vi "Keyence LJ-V7000 Configure.vi"() -> ()   [LabVIEW 2014]
doc: "This example indicates how to change settings of the controller."
uses:
  Public/constant/Comm Interface.ctl
  Public/Clusters/Ethernet Config.ctl
  Public/constant/Setting Depth.ctl
  Public/Clusters/Target Setting.ctl
  Public/constant/Setting Type.ctl
  State Machine State3.ctl
  Keyence LJ-V7000.lvlib
panel:
  out "Accessing \nthe SAVE area":bool
  out "Accessing the SAVE area":bool
  in  "Depth":T1=1 items=["WRITE AREA", "RUNNING AREA", "SAVE AREA"]
  out "Setting Error":u32
  in  "Depth":T1 items=["WRITE AREA", "RUNNING AREA", "SAVE AREA"]
  out "Setting Data":u8[](array[numeric])
  in  "Data Size":u32
  in  "Target Setting":T2={"Type"=1, "Category"=0, "Item"=0, "Target 1"=0, "Target 2"=0, "Target 3"=0, "Target 4"=0} {"Type" items=["ENVIRONMENT"=1, "COMMON MEASUREMENT"=2, "PROGRAM 0"=16, "PROGRAM 1"=17, "PROGRAM 2"=18, "PROGRAM 3"=19, "PROGRAM 4"=20, "PROGRAM 5"=21, "PROGRAM 6"=22, "PROGRAM 7"=23, "PROGRAM 8"=24, "PROGRAM 9"=25, "PROGRAM 10"=26, "PROGRAM 11"=27, "PROGRAM 12"=28, "PROGRAM 13"=29, "PROGRAM 14"=30, "PROGRAM 15"=31]}
  in  "Depth":T1 items=["WRITE AREA", "RUNNING AREA", "SAVE AREA"]
  out "Setting Error":u32
  in  "Setting Data":u8[](array[numeric])
  in  "Target Setting":T2={"Type"=1, "Category"=0, "Item"=0, "Target 1"=0, "Target 2"=0, "Target 3"=0, "Target 4"=0} {"Type" items=["ENVIRONMENT"=1, "COMMON MEASUREMENT"=2, "PROGRAM 0"=16, "PROGRAM 1"=17, "PROGRAM 2"=18, "PROGRAM 3"=19, "PROGRAM 4"=20, "PROGRAM 5"=21, "PROGRAM 6"=22, "PROGRAM 7"=23, "PROGRAM 8"=24, "PROGRAM 9"=25, "PROGRAM 10"=26, "PROGRAM 11"=27, "PROGRAM 12"=28, "PROGRAM 13"=29, "PROGRAM 14"=30, "PROGRAM 15"=31]}
  in  "Depth":T1 items=["WRITE AREA", "RUNNING AREA", "SAVE AREA"]
  in  "Update Write Settings Area":bool
  in  "Reflect Setting":bool
  in  "Get Setting":bool
  in  "Set Setting":bool
  in  "Stop VI":bool
  in  "Ethernet Config":T4={"IP Address"=[192, 168, 0, 1], "Port No"=24691}
  in  "Comm Interface":T5
  # "Reflect Settings in the\nWRITE Settings Area"
  # "Communication Configuration"
  # "Set Setting"
  # "Get Setting"
  # "Update WRITE Settings Area"
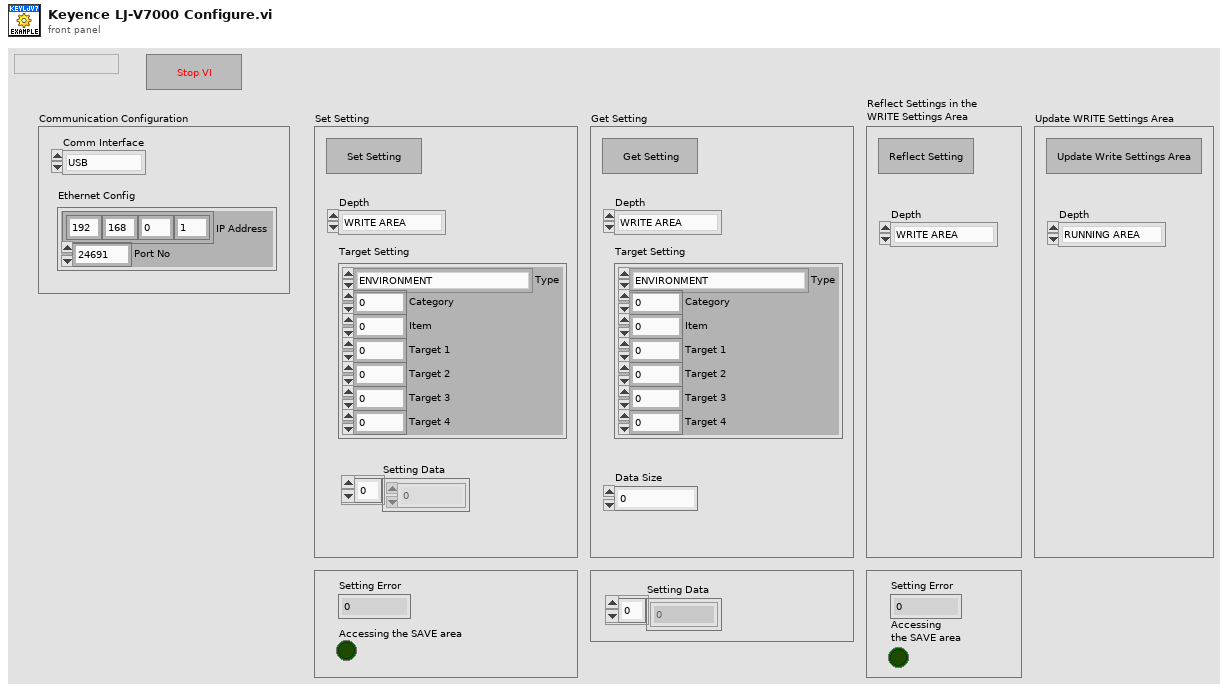
[diagram p1: front panel]
types:
  T1 = typedef "Keyence LJ-V7000.lvlib/Setting Depth.ctl" = u8
  T2 = typedef "Keyence LJ-V7000.lvlib/Target Setting.ctl" = cluster{"Type":T3, "Category":u8, "Item":u8, "Target 1":u8, "Target 2":u8, "Target 3":u8, "Target 4":u8}
  T3 = typedef "Keyence LJ-V7000.lvlib/Setting Type.ctl" = u8
  T4 = typedef "Keyence LJ-V7000.lvlib/Ethernet Config.ctl" = cluster{"IP Address":u8[], "Port No":u16}
  T5 = typedef "Keyence LJ-V7000.lvlib/Comm Interface.ctl" = enum8{"USB", "ETHERNET"}
  T6 = typedef "State Machine State3.ctl" = enum16{"Idle", "Set Setting", "Get Setting", "Reflect Setting", "Update Write Settings Area"}
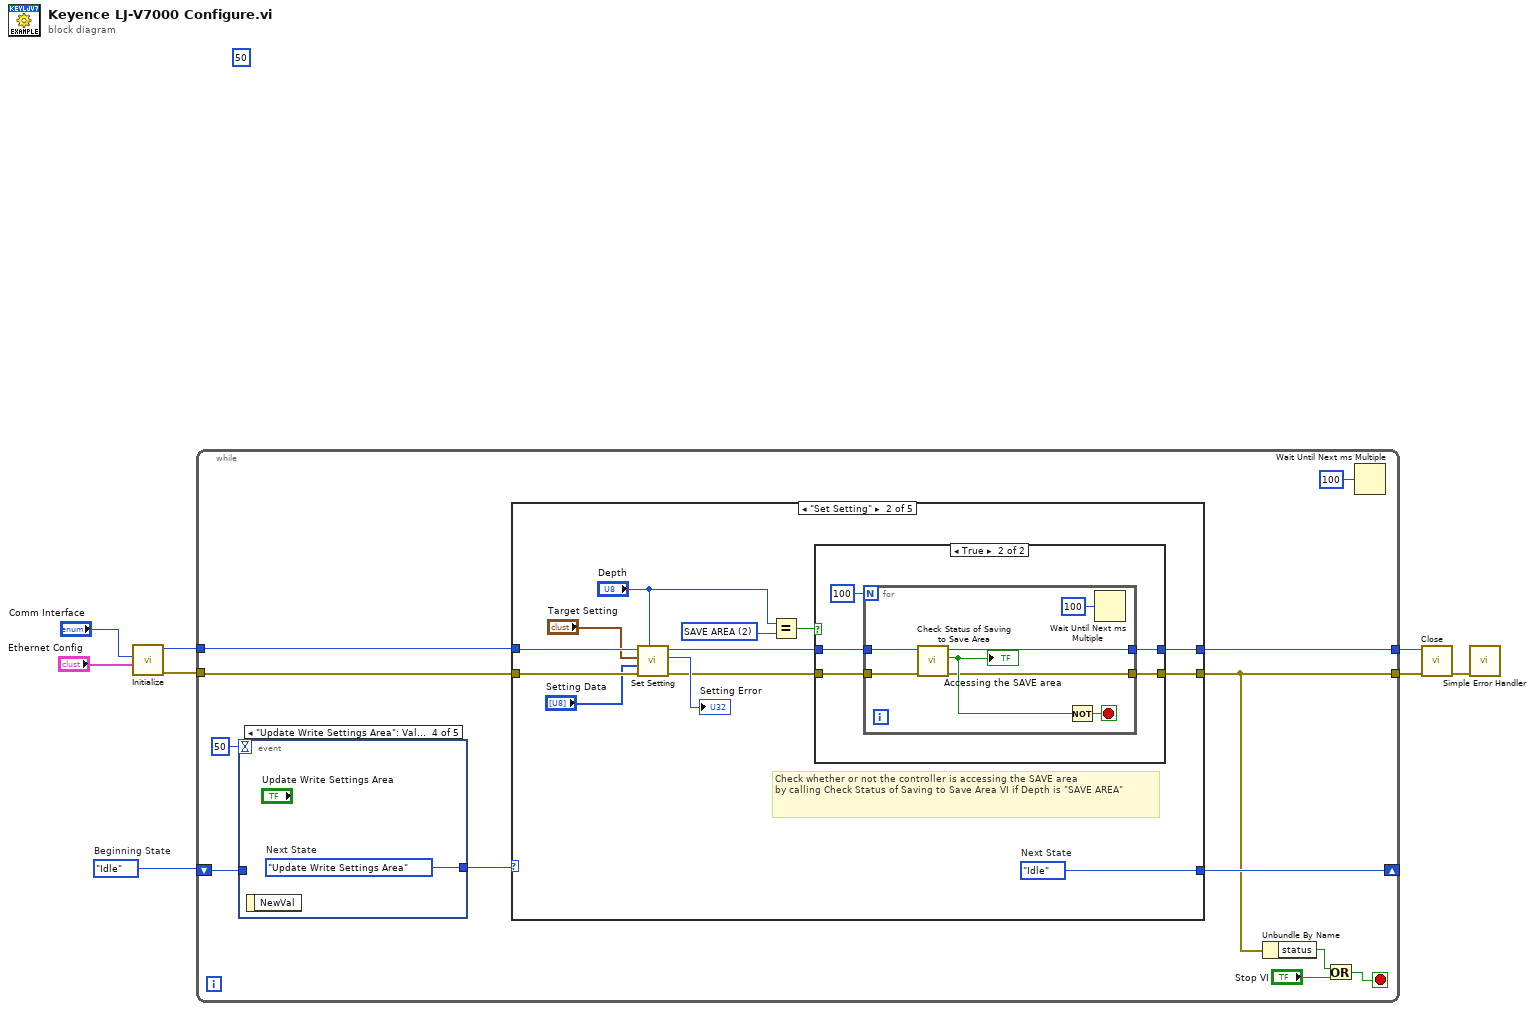
[diagram p0: block diagram]
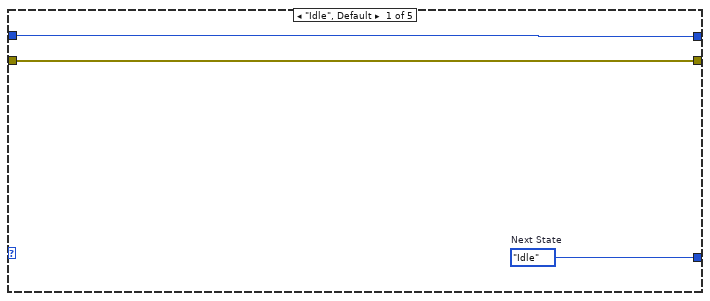
[diagram p2: hidden frame]
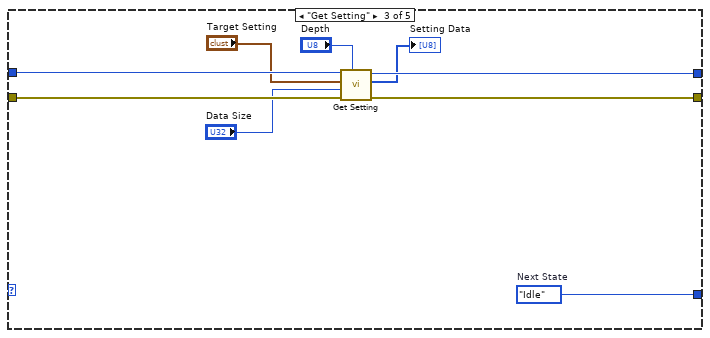
[diagram p4: hidden frame]
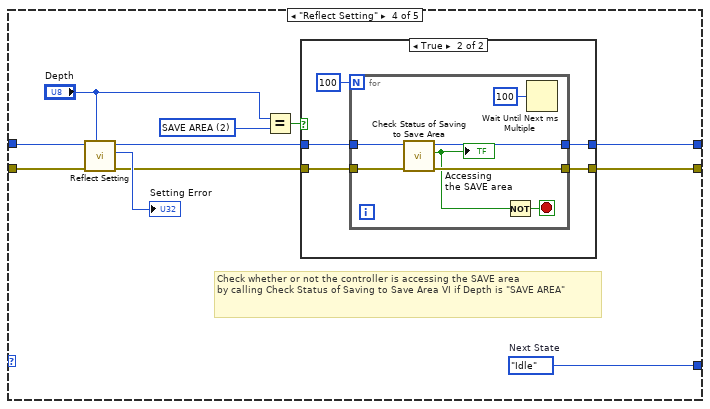
[diagram p5: hidden frame]
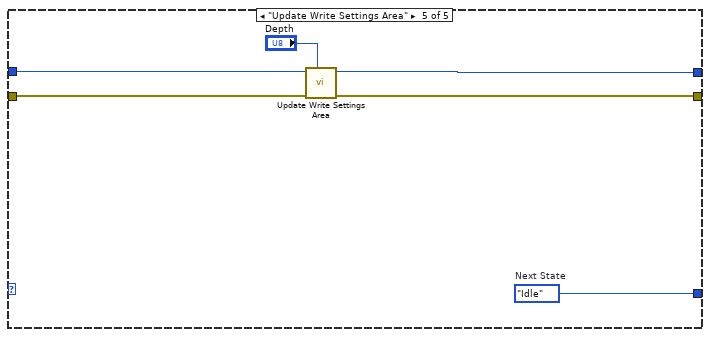
[diagram p7: hidden frame]
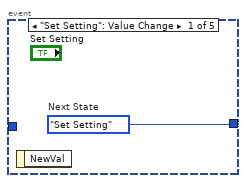
[diagram p8: hidden frame]
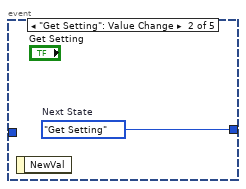
[diagram p9: hidden frame]
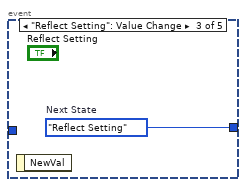
[diagram p10: hidden frame]
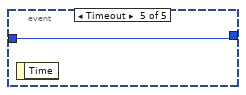
[diagram p11: hidden frame]
diagram:
  w3 = State_Machine_State3."Idle"  # Beginning State
  (unwired) 50
  n1 = call "Initialize.vi"("Ethernet Config"="Ethernet Config", "Comm Interface"="Comm Interface") -> ("error out"=w8:errorcluster, "Device ID out"=w7:i32)  [unwired: 8 in]
  n2 = while {
    shift-right: [w12] -> _
    shift-left: w3 -> [w11]
    tunnel: w8 -> [w15]
    tunnel: w7 -> [w14]
    tunnel: [w9] -> w1
    tunnel: [w13] -> w2
    stop <- w18 stop-if-true
    n3 = event shown="[3] \"Update Write Settings Area\": Value Change" {
      selector: _ -> [_ _ _ _ _]
      dyn-events: _ -> [_ _ _ _ _]
      timeout: 50 -> [_ _ _ _ _]
      tunnel: w11 -> [_ _ _ _ w95]
      tunnel: [w91 w92 w93 w94 w95] -> w16
      event "Set Setting": Value Change {
        w91 = State_Machine_State3."Set Setting"  # Next State
        n4 = event-data() -> ()  [unwired: 1 in, 1 out]
      }
      event "Get Setting": Value Change {
        w92 = State_Machine_State3."Get Setting"  # Next State
        n5 = event-data() -> ()  [unwired: 1 in, 1 out]
      }
      event "Reflect Setting": Value Change {
        w93 = State_Machine_State3."Reflect Setting"  # Next State
        n6 = event-data() -> ()  [unwired: 1 in, 1 out]
      }
      event "Update Write Settings Area": Value Change {
        w94 = State_Machine_State3."Update Write Settings Area"  # Next State
        n7 = event-data() -> ()  [unwired: 1 in, 1 out]
      }
      event Timeout {
        n8 = event-data() -> ()  [unwired: 1 in, 1 out]
      }
    }
    n9 = case shown="\"Set Setting\"" w16 {
      tunnel: w15 -> [w22 w36 w59 w70 w87]
      tunnel: w14 -> [w23 w35 w58 w69 w90]
      tunnel: [w22 w25 w56 w60 w88] -> w9
      tunnel: [w23 w24 w57 w61 w89] -> w13
      tunnel: [w21 w34 w55 w68 w86] -> w12
      frame "Idle", Default {
        w21 = State_Machine_State3."Idle"  # Next State
      }
      frame "Set Setting" {
        w27 = T1 2 items=["WRITE AREA", "RUNNING AREA", "SAVE AREA"] ("Depth 2")
        w34 = State_Machine_State3."Idle"  # Next State
        # "Check whether or not the controller is accessing the SAVE area \nby calling Check Status of Saving to Save Area VI if Depth is \"SAVE AREA\""
        n10 = call "Set Setting.vi"("Depth"="Depth", "error in (no error)"=w36, "Setting Data"="Setting Data", "Target Setting"="Target Setting", "Device ID (0)"=w35) -> ("error out"=w30:errorcluster, "Setting Error"=→"Setting Error":u32, "Device ID out"=w29:i32)  [unwired: 4 in]
        n11 = Equal?(x="Depth", y=w27) -> (x = y?=w28:bool)
        n12 = case shown="True" w28 {
          tunnel: w30 -> [w37 w43]
          tunnel: w29 -> [w38 w42]
          tunnel: [w37 w40] -> w25
          tunnel: [w38 w39] -> w24
          frame False {
          }
          frame True {
            n13 = for {
              N: 100 -> [_]
              tunnel: w43 -> [w50]
              tunnel: w42 -> [w49]
              tunnel: [w45] -> w40
              tunnel: [w44] -> w39
              stop <- w47 stop-if-true
              n14 = call "Check Status of Saving to Save Area.vi"("error in (no error)"=w50, "Device ID (0)"=w49) -> ("error out"=w45:errorcluster, "Busy"=w46:bool, "Device ID out"=w44:i32)  [unwired: 7 in]
              "Accessing the SAVE area" <- w46
              n15 = Not(x=w46) -> (.not. x?=w47:bool)
              n16 = Wait Until Next ms Multiple(millisecond multiple=u32 100 ("ミリ秒倍数")) -> ()  [unwired: 1 out]
            }
          }
        }
      }
      frame "Get Setting" {
        w55 = State_Machine_State3."Idle"  # Next State
        n17 = call "Get Setting.vi"("Depth"="Depth", "error in (no error)"=w59, "Data Size"="Data Size", "Target Setting"="Target Setting", "Device ID (0)"=w58) -> ("error out"=w56:errorcluster, "Setting Data"=→"Setting Data":u8[], "Device ID out"=w57:i32)  [unwired: 4 in]
      }
      frame "Reflect Setting" {
        w64 = T1 2 items=["WRITE AREA", "RUNNING AREA", "SAVE AREA"] ("Depth 2")
        w68 = State_Machine_State3."Idle"  # Next State
        # "Check whether or not the controller is accessing the SAVE area \nby calling Check Status of Saving to Save Area VI if Depth is \"SAVE AREA\""
        n18 = call "Reflect Setting.vi"("Depth"="Depth", "error in (no error)"=w70, "Device ID (0)"=w69) -> ("error out"=w62:errorcluster, "Setting Error"=→"Setting Error":u32, "Device ID out"=w63:i32)  [unwired: 6 in]
        n19 = Equal?(x="Depth", y=w64) -> (x = y?=w66:bool)
        n20 = case shown="True" w66 {
          tunnel: [w71 w76] -> w60
          tunnel: [w72 w75] -> w61
          tunnel: w63 -> [w72 w74]
          tunnel: w62 -> [w71 w73]
          frame False {
          }
          frame True {
            n21 = for {
              N: 100 -> [_]
              tunnel: [w82] -> w76
              tunnel: [w81] -> w75
              tunnel: w74 -> [w80]
              tunnel: w73 -> [w79]
              stop <- w83 stop-if-true
              n22 = call "Check Status of Saving to Save Area.vi"("error in (no error)"=w79, "Device ID (0)"=w80) -> ("error out"=w82:errorcluster, "Busy"=w78:bool, "Device ID out"=w81:i32)  [unwired: 7 in]
              "Accessing \nthe SAVE area" <- w78
              n23 = Not(x=w78) -> (.not. x?=w83:bool)
              n24 = Wait Until Next ms Multiple(millisecond multiple=u32 100 ("ミリ秒倍数")) -> ()  [unwired: 1 out]
            }
          }
        }
      }
      frame "Update Write Settings Area" {
        w86 = State_Machine_State3."Idle"  # Next State
        n25 = call "Update Write Settings Area.vi"("Depth"="Depth", "error in (no error)"=w87, "Device ID (0)"=w90) -> ("error out"=w88:errorcluster, "Device ID out"=w89:i32)  [unwired: 7 in]
      }
    }
    n26 = Unbundle By Name(w9) -> ("status"=w10:bool)
    n27 = Or(x=w10, y="Stop VI") -> (x .or. y?=w18:bool)
    n28 = Wait Until Next ms Multiple(millisecond multiple=u32 100 ("ミリ秒倍数")) -> ()  [unwired: 1 out]
  }
  n29 = call "Close.vi"("error in (no error)"=w1, "Device ID (0)"=w2) -> ("error out"=w6:errorcluster)  [unwired: 8 in, 1 out]
  n30 = call <vilib>:"Simple Error Handler.vi"("error in (no error)"=w6) -> ()  [unwired: 4 in, 5 out]
